vi "Set Install Mode.vi"(8 "error in":errorcluster, 11 "session in":refnum<k21>) -> (0 "error out":errorcluster, 3 "session out":refnum<k21>)   [LabVIEW 2013]
uses:
  <resource>/objmgr/nisysapi.rc
  <vilib>/nisyscfg/nisyscfg.lvlib
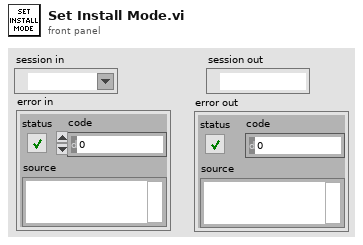
[diagram p1: front panel]
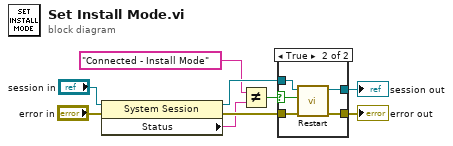
[diagram p0: block diagram]
diagram:
  n1 = property class="System Session"(reference="session in", error in="error in") -> (reference out=w6:refnum<k21>, error out=w8:errorcluster, "Status"=w5:string)
  n2 = Not Equal?(x="Connected - Install Mode" ("y"), y=w5) -> (x != y?=w3:bool)
  n3 = case shown="True" w3 {
    selector: w3 -> [_ w12]
    tunnel: w8 -> [w10 w16]
    tunnel: [w10 w15] -> w2
    tunnel: w6 -> [w11 w14]
    tunnel: [w11 w13] -> w1
    frame False {
    }
    frame True {
      n4 = call <vilib>:"Restart.vi"("error in (no error)"=w16, "install mode (F)"=w12, "session in"=w14) -> ("error out"=w15:errorcluster, "session out"=w13:refnum<k21>)  [unwired: 6 in, 1 out]
    }
  }
  "error out" <- w2
  "session out" <- w1
